vi "Build Variant Look Up Table.vi"(6 "Operations":T1=[{"String"="Equals", "Value"="EQ"}, {"String"="Not Equal", "Value"="NotEQ"}, {"String"="Greater", "Value"="GT"}, {"String"="Greater Than or Equal To", "Value"="GTEQ"}, {"String"="Less Than", "Value"="LT"}, {"String"="Less Than or Equal To", "Value"="LTEQ"}, {"String"="Greater Than Less Than", "Value"="GTLT"}], 8 "error in (no error)":errorcluster, 11 "LUT in":variant) -> (0 "error out":errorcluster, 3 "LUT out":variant)   [LabVIEW 2016]
uses:
  <vilib>/Utility/miscctls.llb/LVComboBoxStrsAndValuesArrayTypeDef.ctl
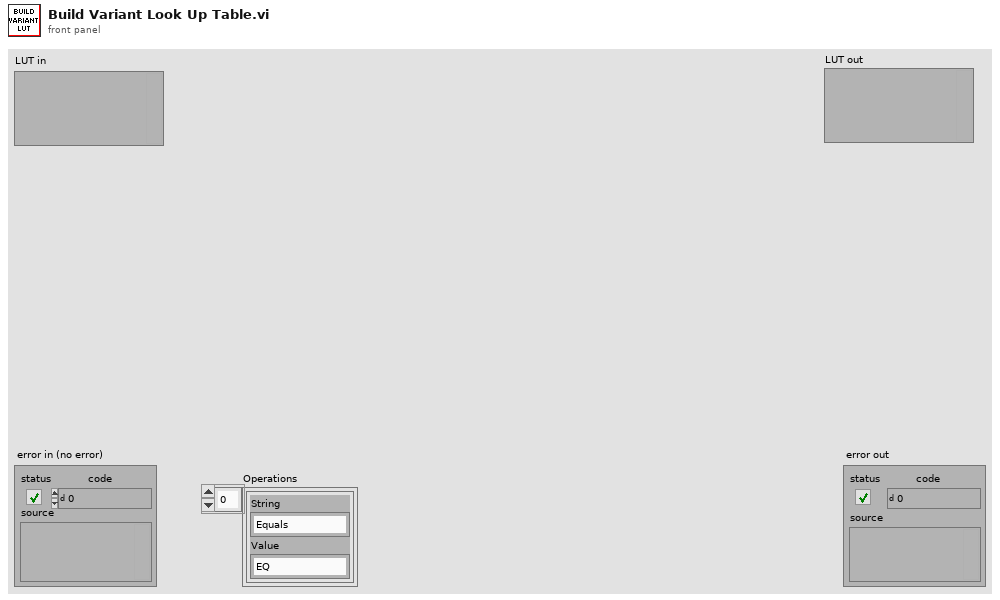
[diagram p1: front panel]
types:
  T1 = typedef "LVComboBoxStrsAndValuesArrayTypeDef.ctl" = cluster{"String":string, "Value":string}[]
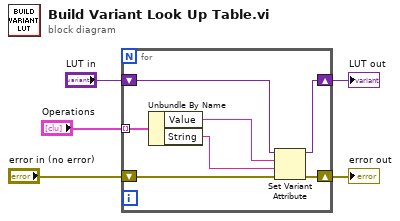
[diagram p0: block diagram]
diagram:
  n1 = for {
    tunnel: "Operations" -> [w12] mode=indexing
    shift-right: [w8] -> w3
    shift-left: "LUT in" -> [w9]
    shift-right: [w6] -> w1
    shift-left: "error in (no error)" -> [w7]
    n2 = Unbundle By Name(w12) -> ("Value"=w11:string, "String"=w10:string)
    n3 = Set Variant Attribute(Variant=w9, name=w11, value=w10, error in=w7) -> (Variant out=w8:variant, error out=w6:errorcluster)  [unwired: 1 out]
  }
  "error out" <- w1
  "LUT out" <- w3
